vi "subGetElapsedTime.vi"(11 "millisecond timer value in":u32) -> (2 "Elapsed time (m)":dbl, 3 "millisecond timer value out":u32)   [LabVIEW 2020, in "DependencyInspector.lvlib"]
uses:
  DependencyInspector.lvlib
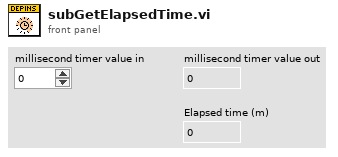
[diagram p1: front panel]
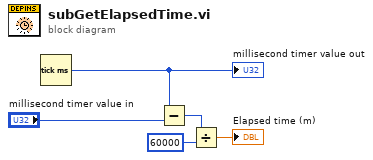
[diagram p0: block diagram]
diagram:
  n1 = Tick Count (ms)() -> (millisecond timer value=w5:u32)
  "millisecond timer value out" <- w5
  n2 = Subtract(x=w5, y="millisecond timer value in") -> (x-y=w2:u32)
  n3 = Divide(x=w2, y=u32 60000) -> (x/y=→"Elapsed time (m)":dbl)
